vi "Publisher.vi"() -> ()   [LabVIEW 2020]
panel:
  in  "stop":bool
  in  "String 2":string
  in  "Numeric 2":dbl format="%#_13g"
  in  "Boolean 2":bool
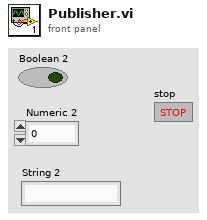
[diagram p1: front panel]
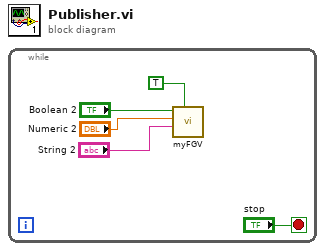
[diagram p0: block diagram]
diagram:
  n1 = while {
    stop <- "stop" stop-if-true
    n2 = call "myFGV.vi"("P/S?"=TRUE, "String 2"="String 2", "Numeric 2"="Numeric 2", "Boolean 2"="Boolean 2") -> ()  [unwired: 5 in, 3 out]
  }
